vi "send arr of complex.vi"() -> ()   [LabVIEW 2018, in "LV-Julia_ZMQ-Roundtrip_lib.lvlib"]
uses:
  LV-Julia_ZMQ-Roundtrip_lib.lvlib
  Julia functions enum.ctl
  example args cluster.ctl
  example server response cluster.ctl
  Server or client state.ctl
  Commands v2.ctl
  commands LV2Jl.ctl
  5d385633-7562-4640-8300-e9530f023818.vi
  c1ad7611-f00e-47ba-b950-502655f00f75.vi
  9ad41121-06aa-4420-b411-b77d699816f6.vi
  cb7a600e-1a3f-45a0-9149-1773accb9ab7.vi
  5d385633-7562-4640-8300-e9530f023818.vi/6859dd59-390a-43a5-80d6-b850cc946908.vi
  c1ad7611-f00e-47ba-b950-502655f00f75.vi/80aec176-b522-404b-8e46-2a0289bb58a0.vi
  c1ad7611-f00e-47ba-b950-502655f00f75.vi/04accb61-e35d-4ab7-b871-c494e33a5348.vi
  c1ad7611-f00e-47ba-b950-502655f00f75.vi/92d51360-c0ee-4ff7-8caf-feee08f8ab08.vi
  9ad41121-06aa-4420-b411-b77d699816f6.vi/d88d09b4-18f7-40f3-adf3-7357a8bfcfb8.vi
  9ad41121-06aa-4420-b411-b77d699816f6.vi/d67fd74d-9395-494a-9148-e10c4998c495.vi
  9ad41121-06aa-4420-b411-b77d699816f6.vi/5b92d6f7-79f3-4f13-bed0-a1e21803906d.vi
  5d385633-7562-4640-8300-e9530f023818.vi/6859dd59-390a-43a5-80d6-b850cc946908.vi/a2dcdd49-0f87-4276-a9fa-9a26cd58d630.vi
  5d385633-7562-4640-8300-e9530f023818.vi/6859dd59-390a-43a5-80d6-b850cc946908.vi/a2dcdd49-0f87-4276-a9fa-9a26cd58d630.vi/68fcb661-db1e-46e4-9d7c-eca83fced4b4.vi
  check ID validity.vi
  bindata_descr to JSON.vi
  convert Jl functions enum to string.vi
  check cluster field names.vi
  concat JSON.vi
panel:
  out "element":sgl
  in  "index to return":cluster{"idx":u16[]}={"idx"=[1, 1, 1]} {"idx" min=1}
  out "appended array":csg[][][](array[numeric]) format="%.2f"
  in  "stop LV only":bool
  out "JSON args":string
  out "LV Client state out":T1
  out "Jl Server state out":T1
  out "size(s)":i32
  out "unsigned byte array":u8[](array[numeric])
  out "short err code":u8
  out "parsed response 2":cluster{"nums":dbl[]}
  in  "go once":bool
  out "JSON out":string
  out "parsed response":T2 {"bin_lng" format="%.0e"}
  out "final error":errorcluster
  out "current error":errorcluster
  out "status":string
  in  "stop":bool
  in  "Arguments":T3={"arg1"=1, "arg2"=3.14}
  in  "fun2call":T4
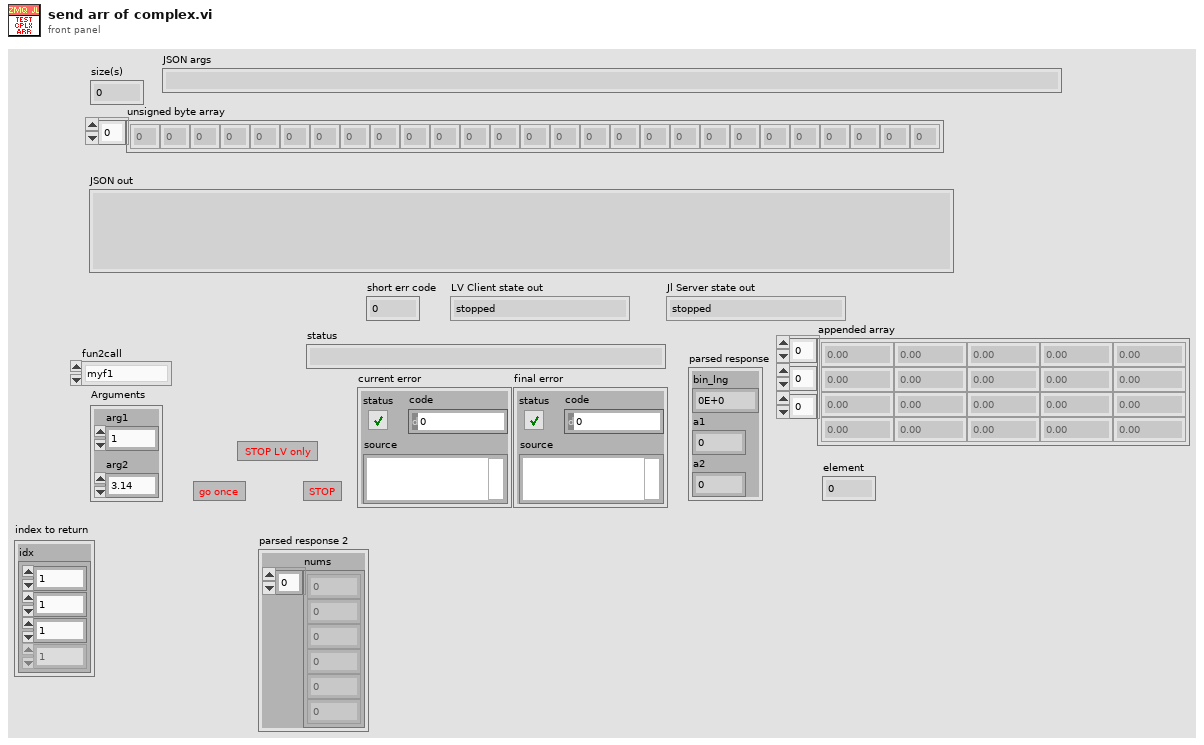
[diagram p1: front panel]
types:
  T1 = typedef "LV-Julia_ZMQ-Roundtrip_lib.lvlib/Server or client state.ctl" = enum16{"stopped", "running", "unknown"}
  T2 = typedef "example server response cluster.ctl" = cluster{"bin_lng":i32, "a1":i32, "a2":dbl}
  T3 = typedef "example args cluster.ctl" = cluster{"arg1":i32, "arg2":dbl}
  T4 = typedef "LV-Julia_ZMQ-Roundtrip_lib.lvlib/Julia functions enum.ctl" = enum16{"myf1", "myf2", "myf3", "test_bin2nums", "test_rgbimg"}
  T5 = typedef "LV-Julia_ZMQ-Roundtrip_lib.lvlib/Commands v2.ctl" = enum16{"Start Jl-server & Init LV-client", "Send request & Get response ", "Stop Jl-server & Cleanup LV-client", "Cleanup LV-client", "Start Jl-server", "Stop Jl-server", "Init LV-Client", "Cleanup LV-Client", "(not allowed)", "Set LV Client state", "Set Jl Server state"}
  T6 = typedef "commands LV2Jl.ctl" = u8
  T7 = typedef "LV-Julia_ZMQ-Roundtrip_lib.lvlib/Bindata description.ctl" = cluster{"nofbytes":i32, "numtype":string, "start":i32, "arrdims":i32[], "kwarg_name":string, "category":string}
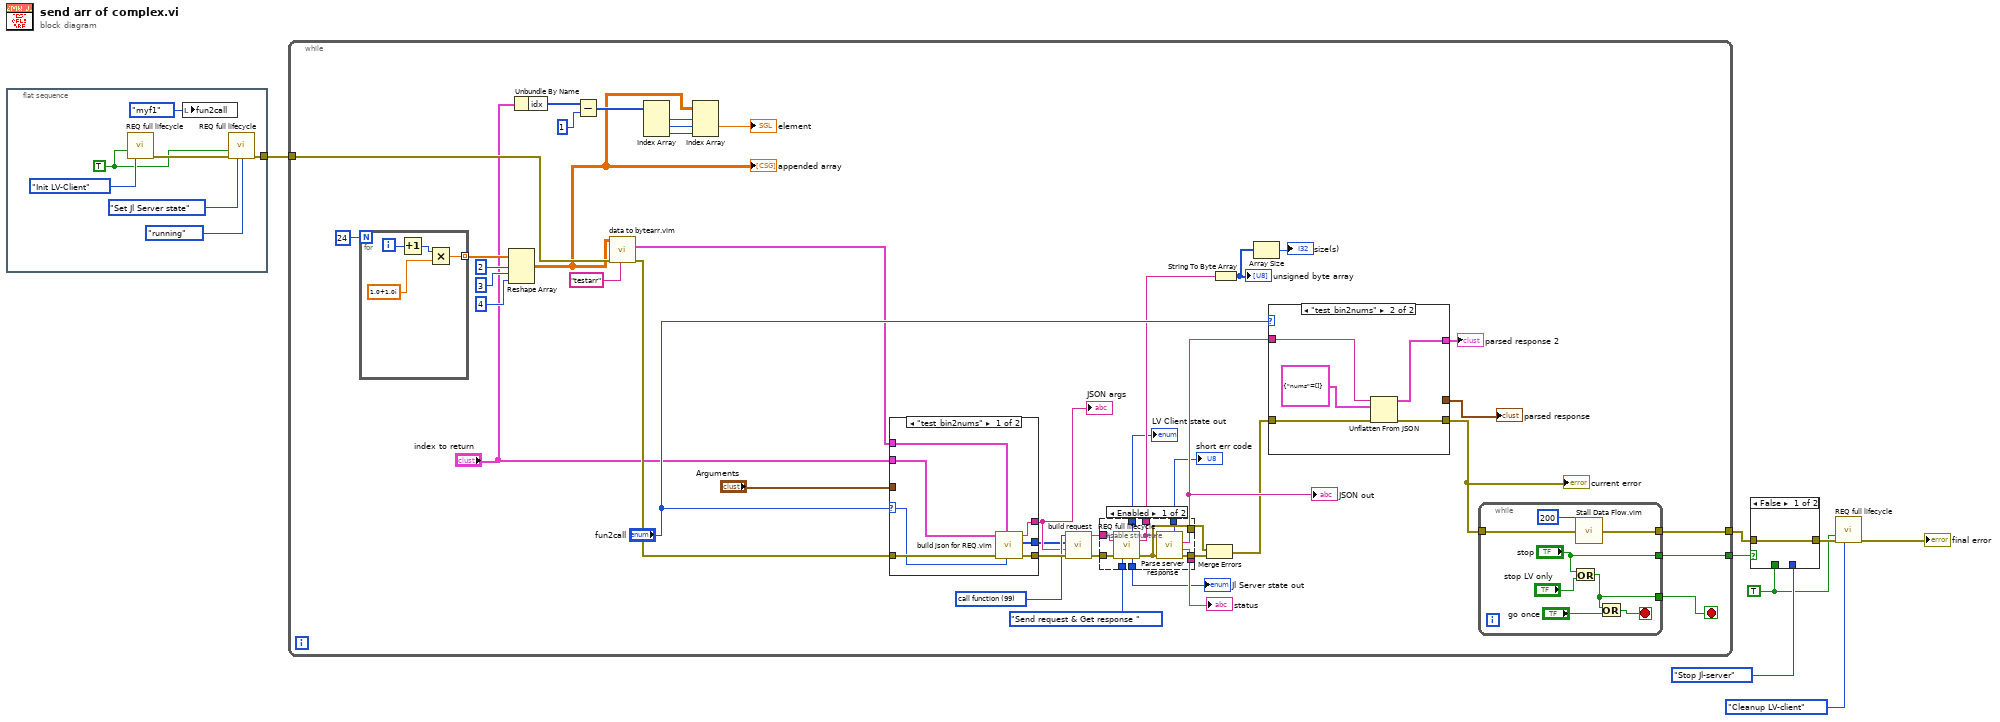
[diagram p0: block diagram]
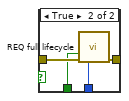
[diagram p2: hidden frame]
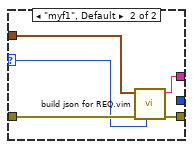
[diagram p4: hidden frame]
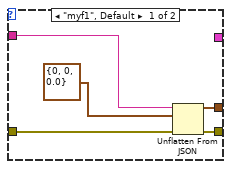
[diagram p5: hidden frame]
diagram:
  w3 = TRUE ("Force command")
  n1 = flat-sequence {
    tunnel: [w13] -> w2
    frame #0 {
      w11 = TRUE ("Force command")
      n2 = call "REQ full lifecycle.vi"("Force command"=w11, "command"=Commands_v2."Init LV-Client") -> ("error out"=w14:errorcluster)  [unwired: 10 in, 3 out]
      n3 = local write "fun2call"(Julia_functions_enum."myf1" ("fun2call")) -> ()
      n4 = call "REQ full lifecycle.vi"("Force command"=w11, "error in"=w14, "command"=Commands_v2."Set Jl Server state", "Jl Server state in"=Server_or_client_state."running") -> ("error out"=w13:errorcluster)  [unwired: 8 in, 3 out]
    }
  }
  n5 = while {
    tunnel: w2 -> [w34]
    tunnel: [w49] -> w8
    tunnel: [w33] -> w1
    stop <- w48 stop-if-true
    w46 = T6 99 items=["call function"=99, "ping"=112, "stop"=115] ("Command")
    n6 = for {
      N: 24 -> [_]
      tunnel: [w62] -> w30 mode=indexing
      i -> [w63]
      n7 = Increment(x=w63) -> (x+1=w61:i32)
      n8 = Multiply(x=w61, y=csg 1.0+1.0i) -> (x*y=w62:csg)
    }
    n9 = Reshape Array(w30, 2 ("dimension size"), 3 ("dimension size"), 4 ("dimension size")) -> (w22:csg[][][])
    "appended array" <- w22
    n10 = Unbundle By Name("index to return") -> ("idx"=w25:u16[])
    n11 = Subtract(x=w25, y=1) -> (x-y=w23:i32[])
    n12 = call "data to bytearr.vim"("kwarg_name"="testarr" ("Tag"), "error in (no error)"=w34, "data in"=w22) -> ("error out"=w42:errorcluster, "Bindata & descr out"=w17:cluster{"bindata_descr":T7[], "bindata":u8[]})  [unwired: 6 in, 1 out]
    n13 = Index Array(array=w23) -> (element #1=w21:i32, element #2=w20:i32, element #3=w19:i32)  [unwired: 3 in]
    n14 = Index Array(array=w22, index (dim 0)=w21, index (dim 1)=w20, index (dim 2)=w19) -> (element=→"element":csg)
    n15 = case shown="\"test_bin2nums\"" "fun2call" {
      selector: "fun2call" -> [w75 w82]
      tunnel: [w80 w85] -> w56
      tunnel: [w79 w84] -> w32
      tunnel: w42 -> [w81 w86]
      tunnel: "Arguments" -> [_ w83]
      tunnel: "index to return" -> [w78 _]
      tunnel: w17 -> [w77 _]
      tunnel: [w76 _] -> w16
      frame "test_bin2nums" {
        n16 = call "build json for REQ.vim"("fun2call"=w75, "Bindata & descr in"=w77, "error in (no error)"=w81, "Arguments 1"=w78) -> ("error out"=w80:errorcluster, "bindata out"=w76:u8[], "JSON string out"=w79:string)  [unwired: 5 in]
      }
      frame "myf1", Default {
        n17 = call "build json for REQ.vim"("fun2call"=w82, "error in (no error)"=w86, "Arguments 1"=w83) -> ("error out"=w85:errorcluster, "JSON string out"=w84:string)  [unwired: 6 in, 1 out]
      }
    }
    "JSON args" <- w32
    n18 = call "build request.vi"("error in (no error)"=w56, "JSON data"=w32, "binary data"=w16, "Command"=w46) -> ("error out"=w54:errorcluster, "REQ string"=w55:string)  [unwired: 6 in]
    n19 = disable-structure shown="Enabled" {
      disable-tunnel: [w74 _] -> w59
      disable-tunnel: [w73 _] -> w58
      disable-tunnel: w55 -> [w72 _]
      disable-tunnel: w54 -> [w71 _]
      disable-tunnel: [w70 _] -> w53
      disable-tunnel: [w69 _] -> w52
      disable-tunnel: Commands_v2."Send request & Get response " ("command") -> [w68 _]
      disable-tunnel: [w67 _] -> w40
      disable-tunnel: [w66 _] -> w39
      disable-tunnel: [w65 _] -> w36
      disable-tunnel: [w64 _] -> w35
      frame Enabled {
        n20 = call "REQ full lifecycle.vi"("data to send"=w72, "error in"=w71, "command"=w68) -> ("LV Client state out"=w64:T1, "server response"=w66:string, "Jl Server state out"=w65:T1, "error out"=w69:errorcluster)  [unwired: 9 in]
        n21 = call "Parse server response.vi"("error in (no error)"=w69, "server response in"=w66) -> ("error out"=w70:errorcluster, "detailed err description"=w74:string, "JSON out"=w73:string, "short err code"=w67:u8)  [unwired: 3 in, 3 out]
      }
      frame Disabled {
      }
    }
    "status" <- w59
    "JSON out" <- w58
    "short err code" <- w40
    "Jl Server state out" <- w36
    "LV Client state out" <- w35
    n22 = Merge Errors(w52, w53) -> (w57:errorcluster)
    n23 = String To Byte Array(string=w39) -> (unsigned byte array=w38:u8[])
    "unsigned byte array" <- w38
    n24 = Array Size(array=w38) -> (size(s)=→"size(s)":i32)
    n25 = case shown="\"test_bin2nums\"" "fun2call" {
      tunnel: w58 -> [w99 w104]
      tunnel: w57 -> [w98 w103]
      tunnel: [w97 w102] -> w50
      tunnel: [w96 _] -> w47
      tunnel: [_ w100] -> w45
      frame "myf1", Default {
        n26 = Unflatten From JSON(JSON string=w99, type and defaults=T2 {"bin_lng"=0, "a1"=0, "a2"=0.0} ("parsed response"), error in (no error)=w98) -> (value=w96:T2, error out=w97:errorcluster)  [unwired: 4 in]
      }
      frame "test_bin2nums" {
        n27 = Unflatten From JSON(JSON string=w104, type and defaults=cluster{"nums":dbl[]} {"nums"=[]} ("parsed response"), error in (no error)=w103) -> (value=w100:cluster{"nums":dbl[]}, error out=w102:errorcluster)  [unwired: 4 in]
      }
    }
    "current error" <- w50
    "parsed response" <- w47
    "parsed response 2" <- w45
    n28 = while {
      tunnel: w50 -> [w94]
      tunnel: [w93] -> w49
      tunnel: [w89] -> w48
      tunnel: ["stop"] -> w33
      stop <- w90 stop-if-true
      n29 = Or(x="stop", y="stop LV only") -> (x .or. y?=w89:bool)
      n30 = call "Stall Data Flow.vim"("value in"=w94, "milliseconds to wait"=u32 200) -> ("value out"=w93:errorcluster)  [unwired: 1 out]
      n31 = Or(x=w89, y="go once") -> (x .or. y?=w90:bool)
    }
  }
  n32 = case shown="False" w1 {
    tunnel: w8 -> [w105 w109]
    tunnel: Commands_v2."Stop Jl-server" ("command") -> [_ w108]
    tunnel: [w105 w107] -> w6
    tunnel: w3 -> [_ w106]
    frame False {
    }
    frame True {
      n33 = call "REQ full lifecycle.vi"("Force command"=w106, "error in"=w109, "command"=w108) -> ("error out"=w107:errorcluster)  [unwired: 9 in, 3 out]
    }
  }
  n34 = call "REQ full lifecycle.vi"("Force command"=w3, "error in"=w6, "command"=Commands_v2."Cleanup LV-client") -> ("error out"=→"final error":errorcluster)  [unwired: 9 in, 3 out]
